vi "filterWfms.vi"(0 "Instrument handle":refnum<k15>, 1 "init/cont (init:F)":bool, 5 "Q factor":i32=2, 7 "F0":dbl format="%.2p", 9 "Order":i32=2, 11 "error in (no error)":errorcluster, 12 "Time signal(s) in":waveform(dbl)[](array[waveform])) -> (4 "Instrument handle out":refnum<k15>, 14 "Filtered time signal(s)":waveform(dbl)[](array[waveform]), 15 "error out":errorcluster)   [LabVIEW 2020]
uses:
  <vilib>/Analysis/3filter.llb/Filter Passband Type.ctl
  <vilib>/Analysis/3filter.llb/Butterworth Filter (DBL).vi
  <vilib>/Analysis/NI_AALBase.lvlib
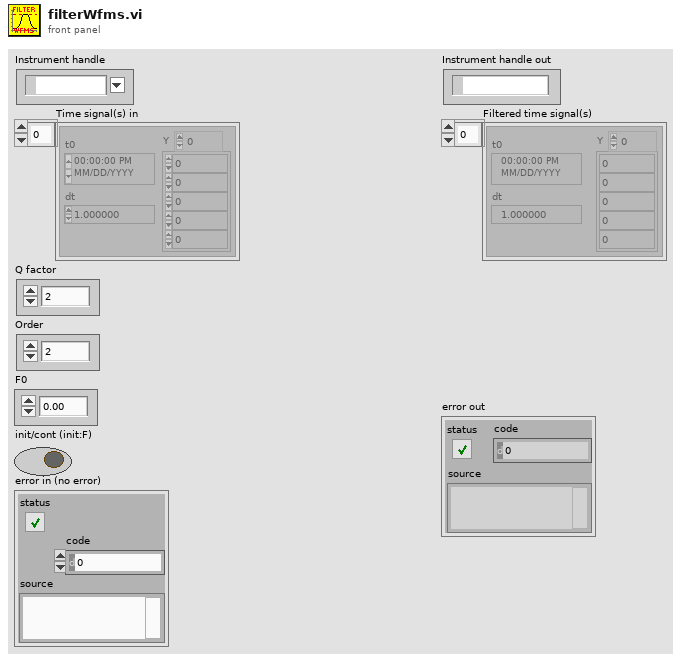
[diagram p1: front panel]
types:
  T1 = typedef "NI_AALBase.lvlib/Filter Passband Type.ctl" = enum32{"Lowpass", "Highpass", "Bandpass", "Bandstop"}
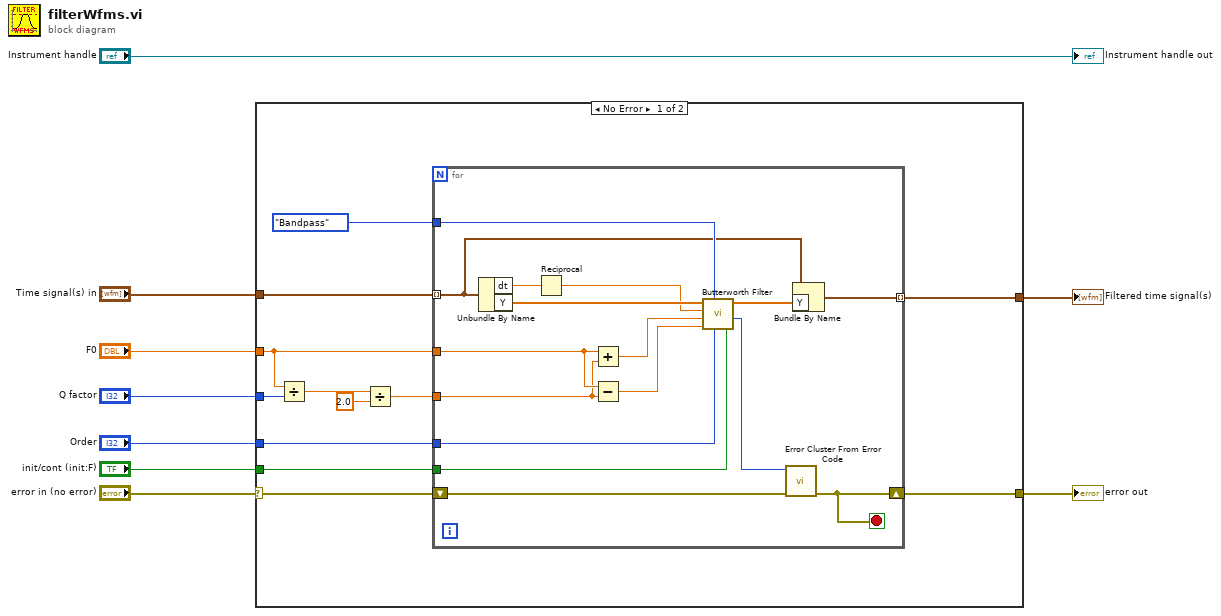
[diagram p0: block diagram]
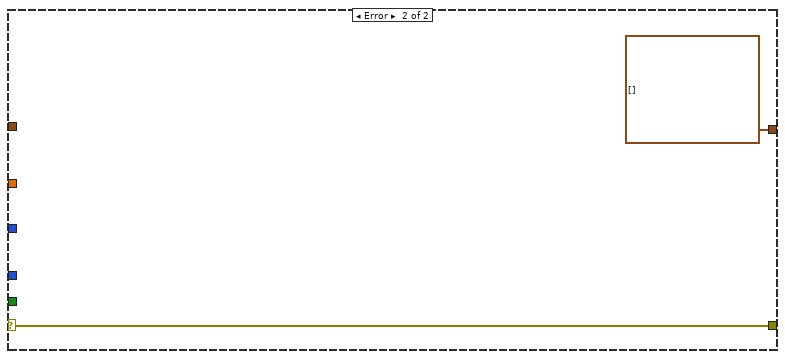
[diagram p2: hidden frame]
diagram:
  n1 = case shown="No Error" "error in (no error)" {
    selector: "error in (no error)" -> [w16 w39]
    tunnel: "Time signal(s) in" -> [w21 _]
    tunnel: "Order" -> [w19 _]
    tunnel: "Q factor" -> [w18 _]
    tunnel: "F0" -> [w17 _]
    tunnel: [w15 w39] -> w3
    tunnel: [w14 waveform(dbl)[] []] -> w4
    tunnel: "init/cont (init:F)" -> [w10 _]
    frame No Error {
      n2 = Divide(x=w17, y=w18) -> (x/y=w13:dbl)
      n3 = Divide(x=w13, y=2.0) -> (x/y=w12:dbl)
      n4 = for {
        tunnel: w21 -> [w24] mode=indexing
        tunnel: Filter_Passband_Type."Bandpass" ("filter type") -> [w37]
        tunnel: w19 -> [w33]
        tunnel: w12 -> [w29]
        tunnel: w17 -> [w30]
        shift-right: [w26] -> w15
        shift-left: w16 -> [w27]
        tunnel: [w23] -> w14 mode=indexing
        tunnel: w10 -> [w22]
        stop <- w26 stop-if-true
        n5 = Unbundle By Name(w24) -> ("dt"=w35:dbl, "Y"=w36:dbl[])
        n6 = Reciprocal(x=w35) -> (1/x=w34:dbl)
        n7 = Add(x=w30, y=w29) -> (x+y=w32:dbl)
        n8 = Subtract(x=w30, y=w29) -> (x-y=w31:dbl)
        n9 = call-poly <vilib>:"Butterworth Filter.vi"("init/cont (init:F)"=w22, "order"=w33, "filter type"=w37, "low cutoff freq: fl"=w31, "high cutoff freq: fh"=w32, "sampling freq: fs"=w34, "X"=w36) -> ("error"=w28:i32, "Filtered X"=w25:dbl[])  [unwired: 1 in]
        n10 = call <vilib>:"Error Cluster From Error Code.vi"("error in (no error)"=w27, "error code (0)"=w28) -> ("error out"=w26:errorcluster)  [unwired: 7 in]
        n11 = Bundle By Name(cluster=w24, "Y"=w25) -> (w23:waveform(dbl))
      }
    }
    frame Error {
    }
  }
  "Filtered time signal(s)" <- w4
  "error out" <- w3
  "Instrument handle out" <- "Instrument handle"
